vi "Concatenate by ref (SubVI).vi"(10 "Response":string, 11 "String ref in":refnum<vi>) -> (3 "String ref off":refnum<vi>)   [LabVIEW 2021]
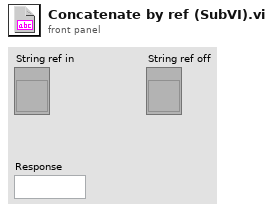
[diagram p1: front panel]
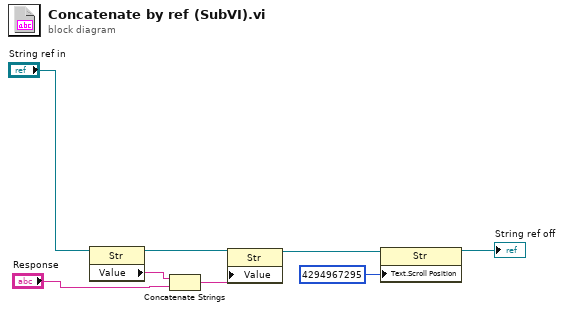
[diagram p0: block diagram]
diagram:
  n1 = property class="Str"(reference="String ref in") -> (reference out=w6:refnum<vi>, "Value"=w5:string)  [unwired: 1 in, 1 out]
  n2 = Concatenate Strings(w5, "Response") -> (w4:string)
  n3 = property class="Str"(reference=w6, "Value"=w4) -> (reference out=w3:refnum<vi>)  [unwired: 1 in, 1 out]
  n4 = property class="Str"(reference=w3, "Text.Scroll Position"=u32 4294967295) -> (reference out=→"String ref off":refnum<vi>)  [unwired: 1 in, 1 out]
